vi "GDSAPI_CreateAttributes.vi"(8 "error in (no error)":errorcluster, 10 "Attributes":T2[](array[typedef]), 11 "ClassPath(*.lvclass)":path) -> (0 "error out":errorcluster, 3 "ClassPathOut(*.lvclass)":path)   [LabVIEW 2016]
doc: "This VI creates Methods in a class."
uses:
  <resource>/Framework/Providers/Open_GDS/ClassProviders/Common/CommonVIs/CommonVIs_AttributeType.ctl
  <resource>/Framework/Providers/Open_GDS/ClassProviders/Common/CommonVIs/CommonVIs_AttributeDataType.ctl
  <resource>/Framework/Providers/Open_GDS/ClassProviders/Common/String/GDSString_AccessScopeModifierType.ctl
  <resource>/Framework/Providers/Open_GDS/ClassProviders/Common/CommonVIs/CommonVIs_ClassNamePathType.ctl
panel:
  in  "Class/TypeDefInfo":T1[](array[typedef])
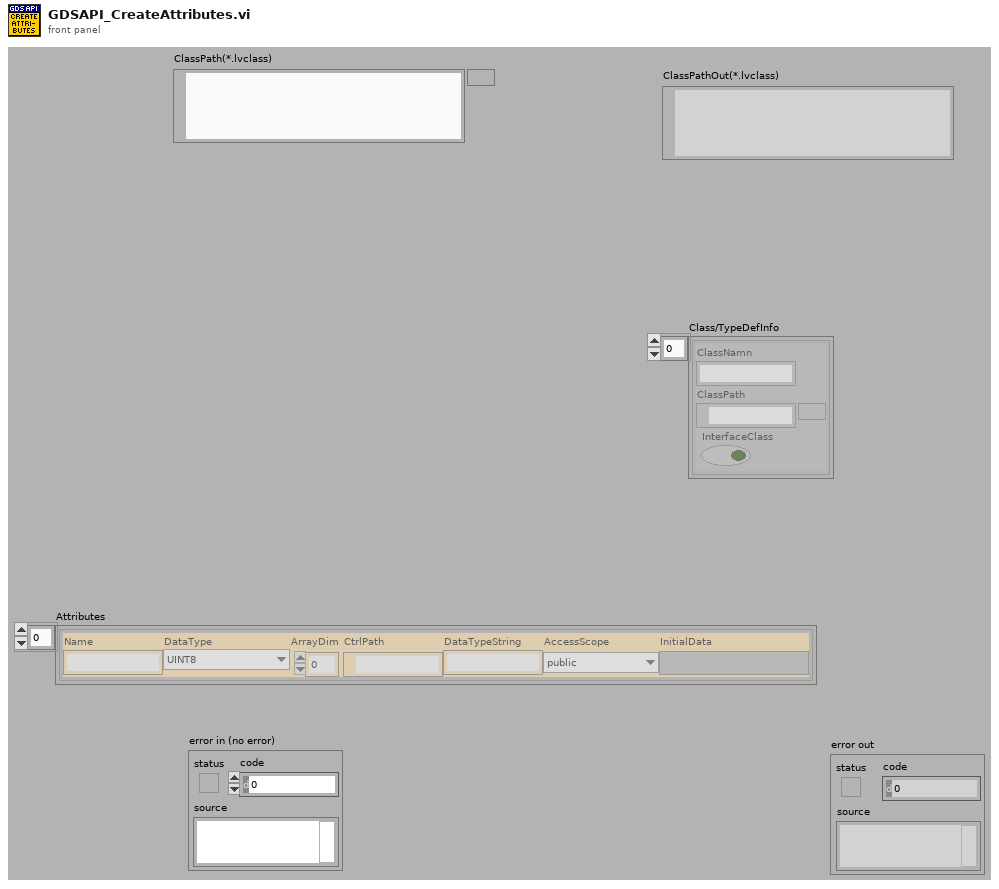
[diagram p1: front panel]
types:
  T1 = typedef "CommonVIs_ClassNamePathType.ctl" = cluster{"ClassNamn":string, "ClassPath":path, "InterfaceClass":bool}
  T2 = typedef "CommonVIs_AttributeType.ctl" = cluster{"Name":string, "DataType":T3, "ArrayDim":i32, "CtrlPath":path, "DataTypeString":string, "AccessScope":T4, "InitialData":variant}
  T3 = typedef "CommonVIs_AttributeDataType.ctl" = enum16{"UINT8", "INT8", "UINT16", "INT16", "UINT32", "INT32", "UINT64", "INT64", "SGL", "DBL", "EXT", "CSG", "CDB", "CXT", "TimeStamp", "STRING", "PATH", "BOOL", "ENUM", "RefNum", "VIRefNum", "LabVIEW Class", "Cluster", "Variant", "TypeDef", "Waveform", "LabVIEW Object", "Other", "void"}
  T4 = typedef "GDSString_AccessScopeModifierType.ctl" = enum16{"public", "private", "protected", "internal"}
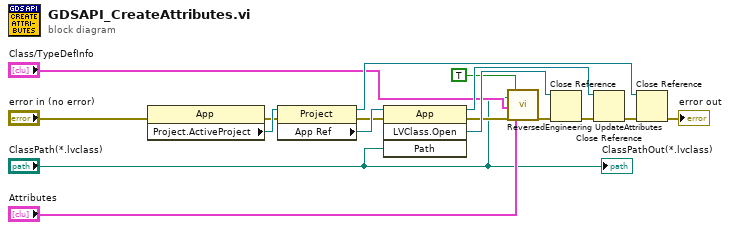
[diagram p0: block diagram]
diagram:
  n1 = property class="App"(error in="error in (no error)") -> (error out=w12:errorcluster, "Project.ActiveProject"=w15:refnum<vi>)  [unwired: 1 in, 1 out]
  n2 = property class="Project"(reference=w15, error in=w12) -> (reference out=w7:refnum<vi>, error out=w13:errorcluster, "App Ref"=w14:refnum<vi>)
  n3 = invoke class="App" method="LVClass.Open"(reference=w14, error in=w13, "Path"="ClassPath(*.lvclass)") -> (reference out=w9:refnum<vi>, error out=w4:errorcluster, "LVClass.Open"=w16:refnum<vi>)  [unwired: 1 in, 1 out]
  n4 = call <resource>:"ReversedEngineering UpdateAttributes.vi"("ClassPath/LvClassRef"="ClassPath(*.lvclass)", "ClassInfo"="Class/TypeDefInfo", "error in (no error)"=w4, "Don't Prompt (False)"=TRUE, "Attributes"="Attributes") -> ("error out"=w3:errorcluster)  [unwired: 12 in, 2 out]
  n5 = Close Reference(reference=w16, error in (no error)=w3) -> (error out=w10:errorcluster)
  n6 = Close Reference(reference=w9, error in (no error)=w10) -> (error out=w8:errorcluster)
  n7 = Close Reference(reference=w7, error in (no error)=w8) -> (error out=→"error out":errorcluster)
  "ClassPathOut(*.lvclass)" <- "ClassPath(*.lvclass)"
